vi "Fitting test2.vi"(0 "Input Array":dbl[](array[numeric]), 5 "Nb Pixel":dbl, 11 "error in (no error)":errorcluster) -> (4 "Best fit parameters":dbl[](array[numeric]), 6 "Residue":dbl format="%#_13g", 8 "Best fit":dbl[](array[numeric]), 10 "Waveform 2":waveform(dbl), 14 "Covariance":dbl[][](array[numeric]), 15 "error out":errorcluster)   [LabVIEW 2014]
uses:
  <vilib>/gmath/NI_Gmath.lvlib
  <vilib>/gmath/NumericalOptimization/Nonlinear Curve Fit LM formula string.vi
  <vilib>/Analysis/NI_AALPro.lvlib
panel:
  out "Best nonlinear fit":dbl[](array[numeric])
  out "Waveform":waveform(dbl)
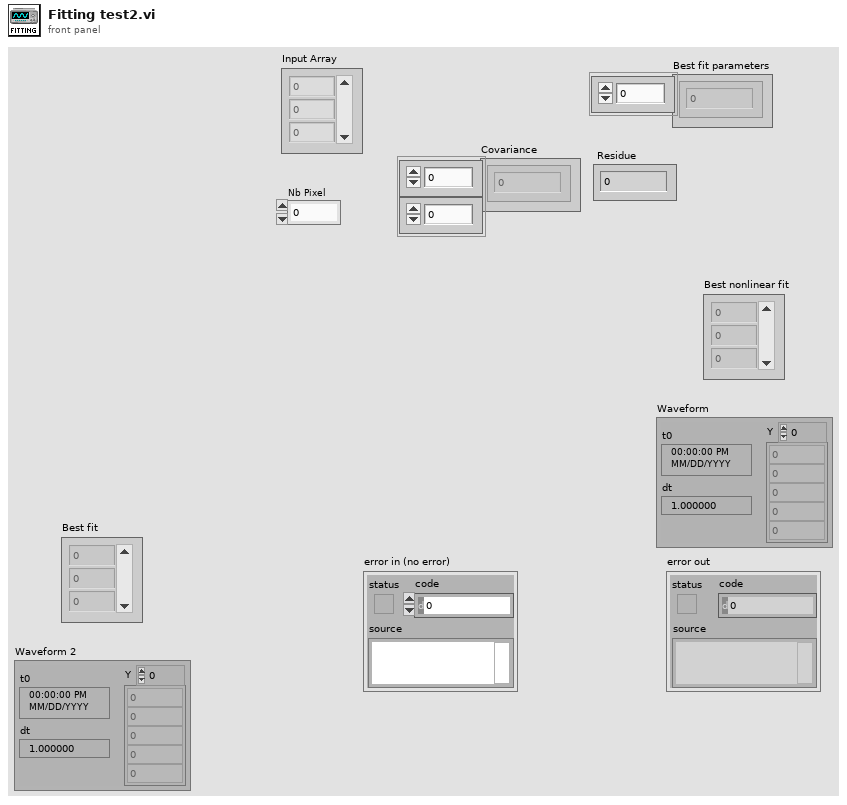
[diagram p1: front panel]
types:
  T1 = cluster{"model":string, "Parameters":string[], "x":string}
  T2 = typedef "NI_Matrix.lvlib/RealMatrix.ctl" = dbl[][]
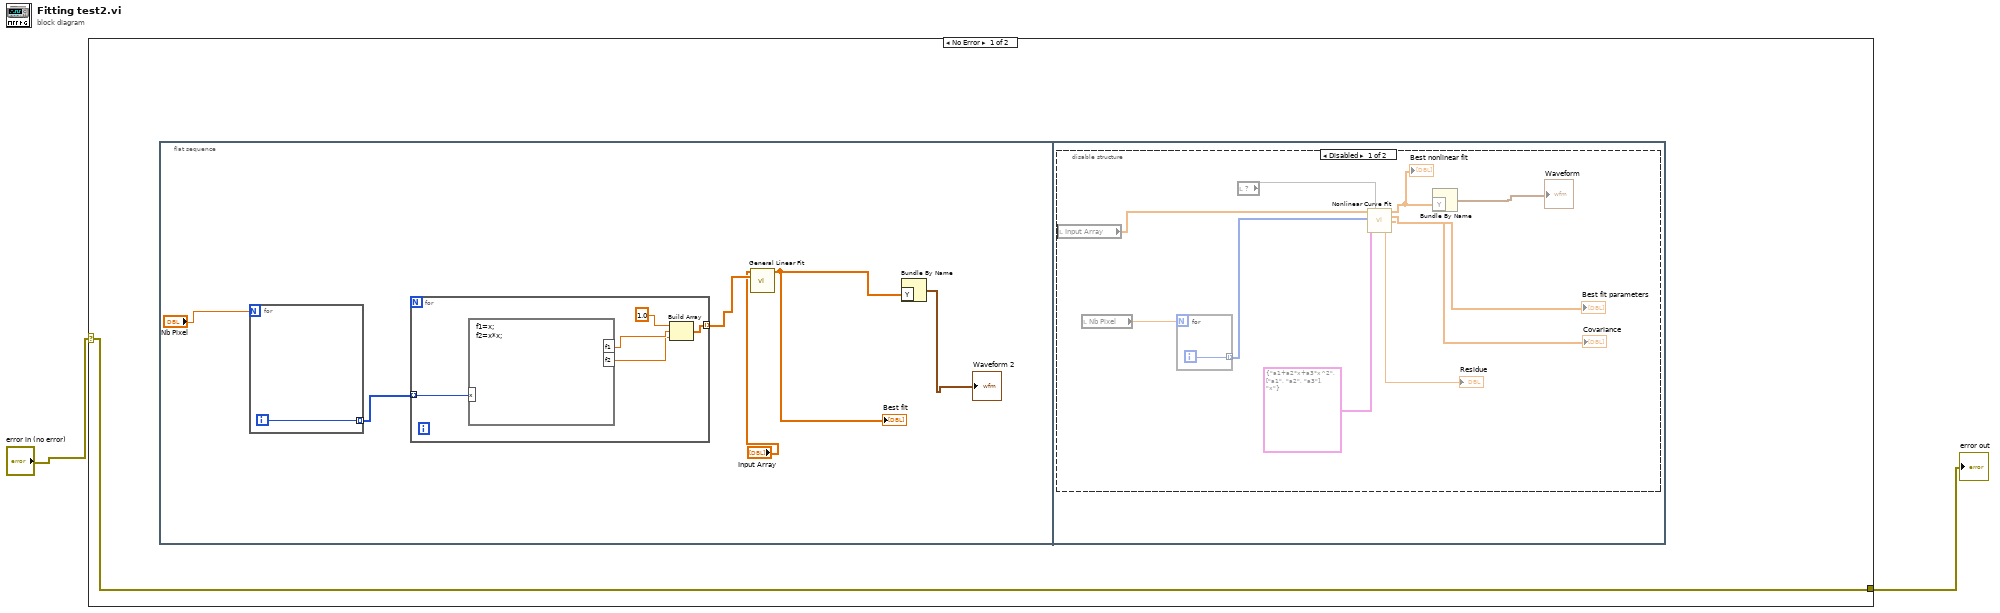
[diagram p0: block diagram]
diagram:
  n1 = case shown="No Error" "error in (no error)" {
    selector: "error in (no error)" -> [w3 w27]
    tunnel: [w3 w27] -> w1
    frame No Error {
      n2 = flat-sequence {
        frame #0 {
          n3 = for {
            N: "Nb Pixel" -> [_]
            tunnel: [w10] -> w6 mode=indexing
            i -> [w10]
          }
          n4 = for {
            tunnel: [w13] -> w7 mode=indexing
            tunnel: w6 -> [w12] mode=indexing
            n5 = formula code="f1=x;\nf2=x*x;"("x"=w12) -> ("f1"=w14:dbl, "f2"=w11:dbl)
            n6 = Build Array(1.0 ("element"), w14, w11) -> (w13:dbl[])
          }
          n7 = call <vilib>:"General Linear Fit.vi"("Y"="Input Array", "H"=w7) -> ("Best Fit"=w4:dbl[])  [unwired: 8 in, 5 out]
          "Best fit" <- w4
          n8 = Bundle By Name("Y"=w4) -> (→"Waveform 2":waveform(dbl))  [unwired: 1 in]
        }
        frame #1 {
          n9 = disable-structure shown="Disabled" {
            frame Disabled {
              n10 = local read "Input Array"() -> (w24:dbl[])
              n11 = local read "Nb Pixel"() -> (w25:dbl)
              n12 = for {
                N: w25 -> [_]
                tunnel: [w26] -> w21 mode=indexing
                i -> [w26]
              }
              n13 = local read item#-1() -> (w16)
              n14 = call-poly <vilib>:"Nonlinear Curve Fit.vi"("Y"=w24, "initial parameters"=w16, "X"=w21, "model description"=T1 {"model"="a1+a2*x+a3*x^2", "Parameters"=["a1", "a2", "a3"], "x"="x"}) -> ("best nonlinear fit"=w23:dbl[], "best fit parameters"=→"Best fit parameters":dbl[], "covariance"=→"Covariance":T2, "residue"=→"Residue":dbl)  [unwired: 7 in, 1 out]
              "Best nonlinear fit" <- w23
              n15 = Bundle By Name("Y"=w23) -> (→"Waveform":waveform(dbl))  [unwired: 1 in]
            }
            frame Enabled {
            }
          }
        }
      }
    }
    frame Error {
    }
  }
  "error out" <- w1
